vi "LocalClient.vi"(6 "timeout (ms) [500]":i32=500, 8 "error in (no error)":errorcluster, 9 "params":variant, 10 "Command in":string, 11 "Instrument in":refnum<class "Instrument.lvclass">) -> (0 "error out":errorcluster, 1 "Data out":variant, 2 "Command out":string, 3 "Instrument out":refnum<class "Instrument.lvclass">)   [LabVIEW 2019, in "Instrument.lvclass"]
doc: "Send a message to a local Instrument process. This VI is basically a wrapper for Instrument.sendMessageToProcess.vi with a mailbox to receive responses.\n\n<b>Command in</b> is a String. Conversion from Enum needs to be handled before calling this method (Use \"Enum to String.vi\")\n\n<b>Data in</b> is a Variant containing your data payload.\n\n<b>Data out</b> is a Variant."
uses:
  Instrument.lvclass
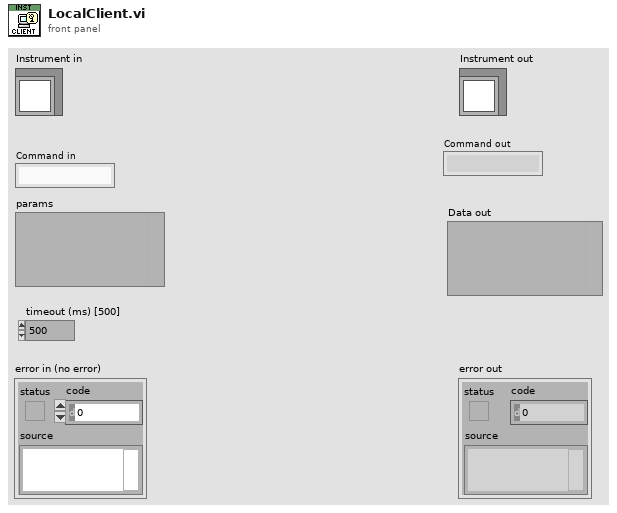
[diagram p1: front panel]
types:
  T1 = typedef "Instrument.lvclass/PublicEvents--Cluster.ctl" = cluster{"MessageFromProcess":refnum<user-event>}
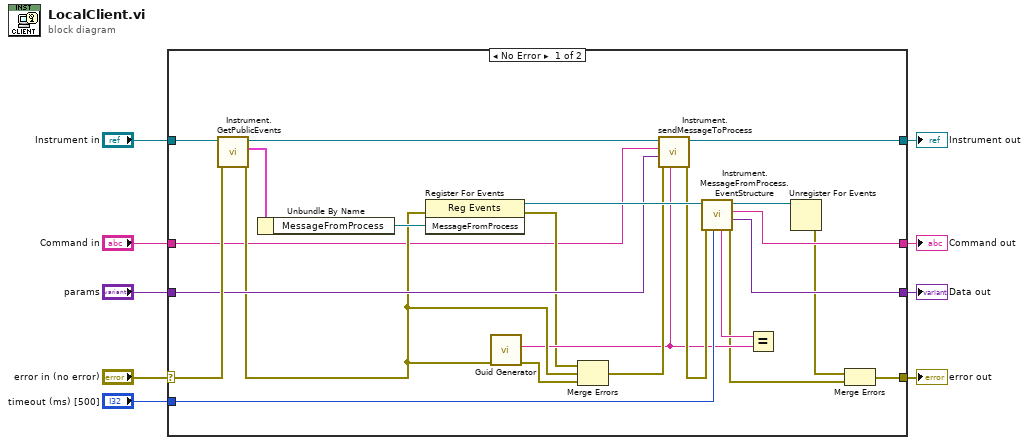
[diagram p0: block diagram]
diagram:
  n1 = case shown="No Error" "error in (no error)" {
    selector: "error in (no error)" -> [w26 w36]
    tunnel: [w10 w36] -> w8
    tunnel: [w32 w35] -> w6
    tunnel: "Instrument in" -> [w28 w35]
    tunnel: "Command in" -> [w15 w34]
    tunnel: "params" -> [w19 w33]
    tunnel: "timeout (ms) [500]" -> [w21 _]
    tunnel: [w14 w34] -> w2
    tunnel: [w13 w33] -> w1
    frame No Error {
      n2 = call "Instrument.GetPublicEvents.vi"("error in (no error)"=w26, "Instrument"=w28) -> ("error out"=w18:errorcluster, "Instrument Public Events"=w31:T1, "Instrument out"=w27:refnum<class "Instrument.lvclass">)  [unwired: 7 in]
      n3 = Unbundle By Name(w31) -> ("MessageFromProcess"=w30:refnum<user-event>)
      n4 = register-events(error in=w18, w30) -> (reference out=w29:refnum<event-registration>, error out=w16:errorcluster)  [unwired: 1 in]
      n5 = call <vilib>:"Guid Generator.vi"("error in (no error)"=w18) -> ("error out"=w20:errorcluster, "GUID"=w17:string)  [unwired: 9 in]
      n6 = Merge Errors(w16, w18, w20) -> (w24:errorcluster)
      n7 = call "Instrument.sendMessageToProcess.vi"("ID"=w17, "error in (no error)"=w24, "Data"=w19, "Command"=w15, "Instrument"=w27) -> ("error out"=w23:errorcluster, "Instrument out"=w32:refnum<class "Instrument.lvclass">)  [unwired: 5 in]
      n8 = call "Instrument.MessageFromProcess.EventStructure.vi"("timeout (ms) [500]"=w21, "error in (no error)"=w23, "Event Registration Refnum in"=w29) -> ("error out"=w12:errorcluster, "Data"=w13:variant, "Command"=w14:string, "Event Registration Refnum out"=w25:refnum<event-registration>, "ID"=w22:string)  [unwired: 4 in]
      n9 = Equal?(x=w22, y=w17) -> ()  [unwired: 1 out]
      n10 = Unregister For Events(event registration refnum=w25) -> (error out=w11:errorcluster)  [unwired: 1 in]
      n11 = Merge Errors(w11, w12) -> (w10:errorcluster)
    }
    frame Error {
      # "leave unwired,\notherwise malleable VI\nwon't adapt properly"
    }
  }
  "error out" <- w8
  "Instrument out" <- w6
  "Command out" <- w2
  "Data out" <- w1
